vi "BRig_RT__Case_Exp__State_initTrial__LC.vi"(0 "input_L_OnOff":u16, 1 "input_L_Block":u16, 2 "input_L_Count":u16, 3 "input_L_Prob":u16, 4 "input_L_Tdelay":u16, 5 "input_L_delayOpt":u16, 6 "input_T_state":u16, 8 "input_iSpout":u16, 10 "input_iTrial_relative":u16, 12 "input_L_T":u16) -> (15 "output_LC_Event":bool, 16 "output_LC_Laser":bool, 18 "output_L_Tstart":u16, 19 "output_L_Tend":u16)   [LabVIEW 2014]
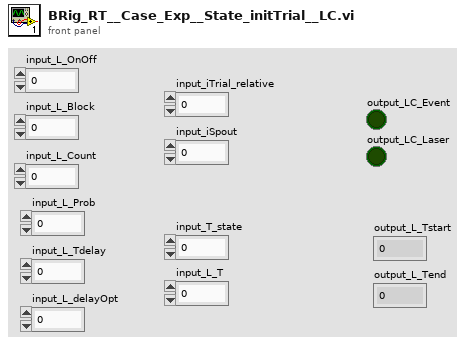
[diagram p1: front panel]
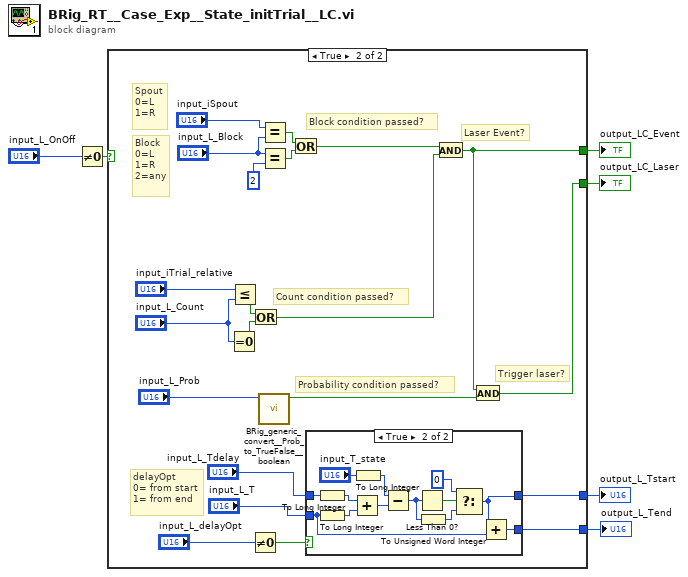
[diagram p0: block diagram]
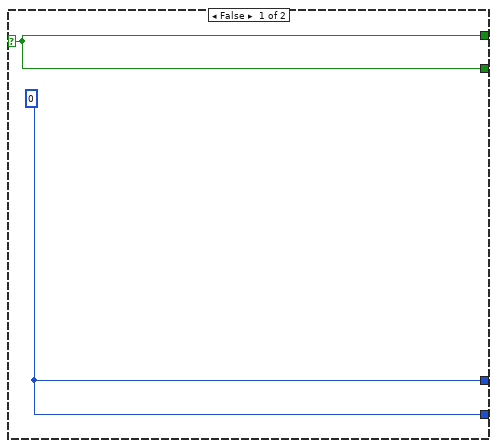
[diagram p2: hidden frame]
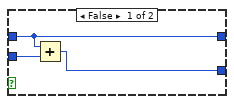
[diagram p3: hidden frame]
diagram:
  n1 = Not Equal To 0?(x="input_L_OnOff") -> (x != 0?=w5:bool)
  n2 = case shown="True" w5 {
    selector: w5 -> [w8 _]
    tunnel: [w8 w16] -> w4
    tunnel: [w8 w15] -> w3
    tunnel: [w7 w10] -> w2
    tunnel: [w7 w9] -> w1
    frame False {
      w7 = u16 0 ("t")
    }
    frame True {
      # "delayOpt\n0= from start\n1= from end"
      # "Trigger laser?"
      # "Laser Event?"
      # "Probability condition passed?"
      # "Count condition passed?"
      # "Block condition passed?"
      # "Spout\n0=L\n1=R"
      # "Block\n0=L\n1=R\n2=any"
      n3 = Equal To 0?(x="input_L_Count") -> (x = 0?=w21:bool)
      n4 = Less Or Equal?(x="input_iTrial_relative", y="input_L_Count") -> (x <= y?=w22:bool)
      n5 = Not Equal To 0?(x="input_L_delayOpt") -> (x != 0?=w13:bool)
      n6 = Or(x=w22, y=w21) -> (x .or. y?=w18:bool)
      n7 = call "BRig_generic_convert__Prob_to_TrueFalse__boolean.vi"("input_probability_u16"="input_L_Prob") -> ("output_TF"=w17:bool)  [unwired: 10 in]
      n8 = Equal?(x="input_iSpout", y="input_L_Block") -> (x = y?=w29:bool)
      n9 = Equal?(x="input_L_Block", y=u16 2) -> (x = y?=w28:bool)
      n10 = Or(x=w29, y=w28) -> (x .or. y?=w19:bool)
      n11 = case shown="True" w13 {
        tunnel: [w30 w33] -> w10
        tunnel: [w32 w34] -> w9
        tunnel: "input_L_T" -> [w31 w35]
        tunnel: "input_L_Tdelay" -> [w30 w45]
        frame False {
          n12 = Add(x=w30, y=w31) -> (x+y=w32:u16)
        }
        frame True {
          n13 = To Long Integer(number=w45) -> (32bit integer=w43:i32)
          n14 = To Long Integer(number=w35) -> (32bit integer=w42:i32)
          n15 = Add(x=w43, y=w42) -> (x+y=w41:i32)
          n16 = To Long Integer(number="input_T_state") -> (32bit integer=w40:i32)
          n17 = Subtract(x=w40, y=w41) -> (x-y=w37:i32)
          n18 = Less Than 0?(x=w37) -> (x < 0?=w39:bool)
          n19 = To Unsigned Word Integer(number=w37) -> (unsigned 16bit integer=w36:u16)
          n20 = Select(t=u16 0, s=w39, f=w36) -> (s? t:f=w33:u16)
          n21 = Add(x=w33, y=w35) -> (x+y=w34:u16)
        }
      }
      n22 = And(x=w19, y=w18) -> (x .and. y?=w16:bool)
      n23 = And(x=w16, y=w17) -> (x .and. y?=w15:bool)
    }
  }
  "output_LC_Event" <- w4
  "output_LC_Laser" <- w3
  "output_L_Tstart" <- w2
  "output_L_Tend" <- w1
